vi "Open Front Panel.vi"(8 "error in (no error)":errorcluster, 11 "Mag Lab Root in":refnum<class "Mag Lab Root.lvclass">) -> (0 "error out":errorcluster, 3 "Mag Lab Root out":refnum<class "Mag Lab Root.lvclass">)   [LabVIEW 2015, in "Mag Lab Root.lvclass"]
uses:
  Mag Lab Root.lvclass
  Mag Lab Root.lvclass/Mag Lab Root.ctl
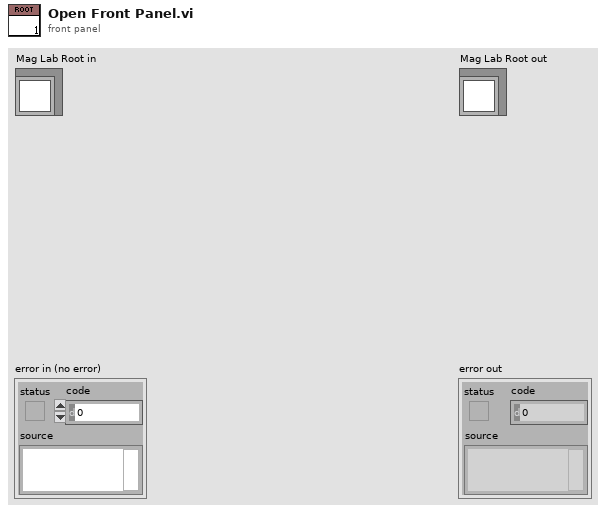
[diagram p1: front panel]
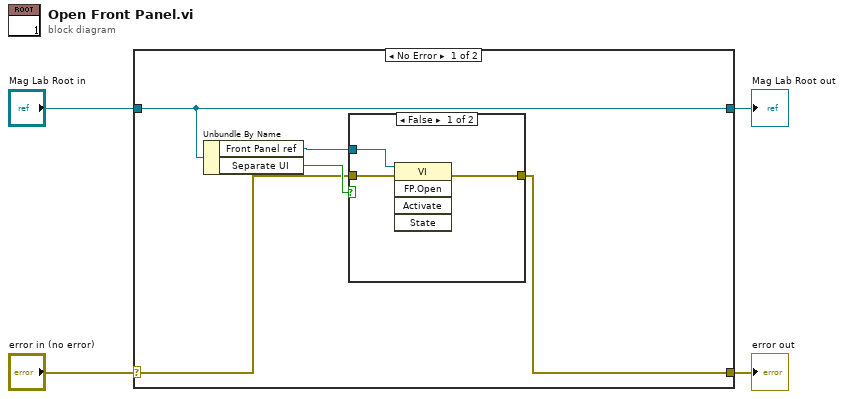
[diagram p0: block diagram]
diagram:
  n1 = case shown="No Error" "error in (no error)" {
    selector: "error in (no error)" -> [w6 w15]
    tunnel: [w5 w15] -> w3
    tunnel: [w7 w14] -> w1
    tunnel: "Mag Lab Root in" -> [w7 w14]
    frame No Error {
      n2 = Unbundle By Name(w7) -> ("Front Panel ref"=w9:refnum<vi>, "Separate UI"=w8:bool)
      n3 = case shown="False" w8 {
        tunnel: w9 -> [w12 _]
        tunnel: w6 -> [w11 w13]
        tunnel: [w10 w13] -> w5
        frame False {
          n4 = invoke class="VI" method="FP.Open"(reference=w12, error in=w11) -> (error out=w10:errorcluster)  [unwired: 3 in, 4 out]
        }
        frame True {
        }
      }
    }
    frame Error {
    }
  }
  "error out" <- w3
  "Mag Lab Root out" <- w1
